vi "Instr_InitObject.vi"(8 "error in (no error)":errorcluster, 9 "Instrument Configuration":variant, 10 "GPIB Address":string, 11 "LXIPXISwitching in":refnum<class "LXIPXISwitching.lvclass">) -> (0 "error out":errorcluster, 3 "LXIPXISwitching out":refnum<class "LXIPXISwitching.lvclass">)   [LabVIEW 2018, in "LXIPXISwitching.lvclass"]
uses:
  LXIPXISwitching.lvclass
  LXIPXISwitching.lvclass/LXIPXISwitching.ctl
  InstrumentSetup.vi
  InstrControl.lvclass
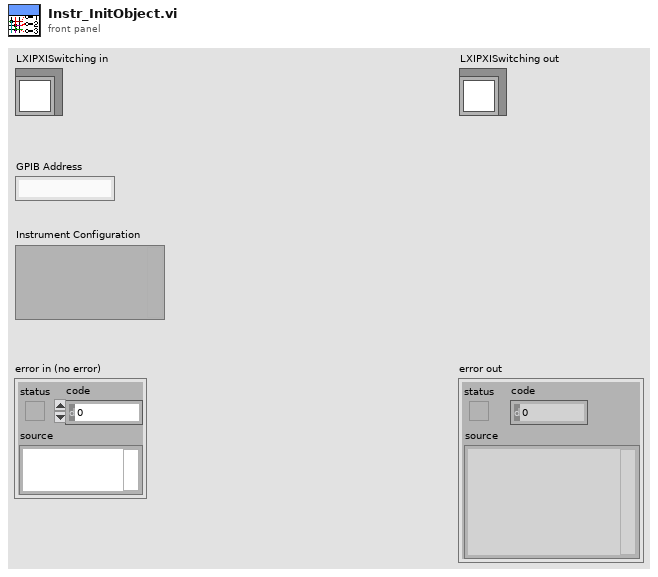
[diagram p1: front panel]
types:
  T1 = cluster{"MUX ":string, "Matrix":string, "Breadboard":string, "MUX  PN":string, "Matrix PN":string, "Breadboard PN":string}
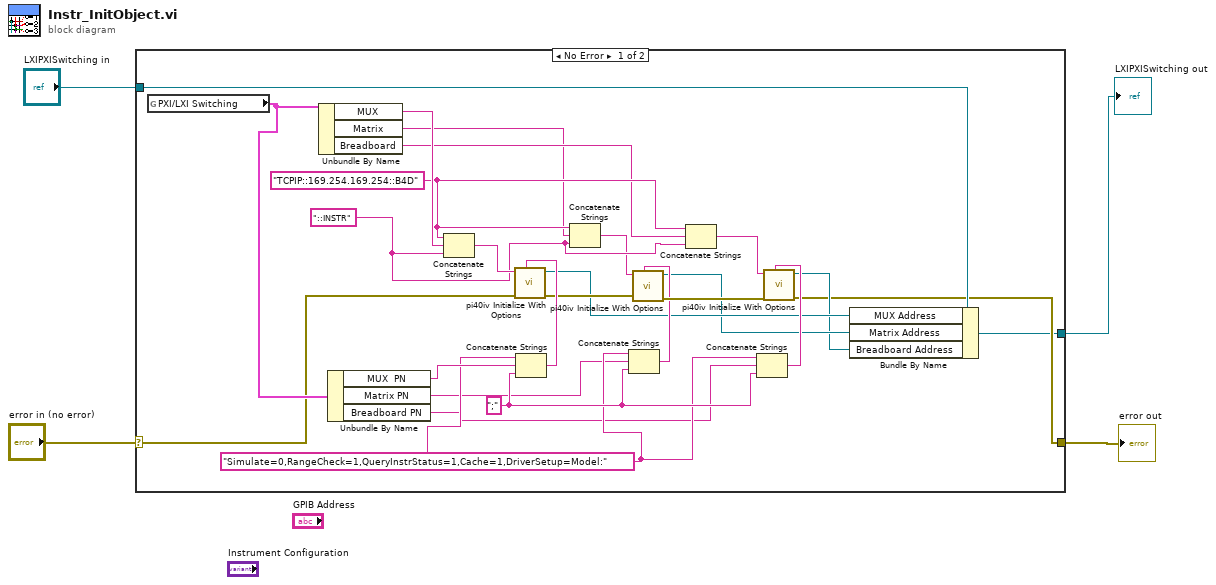
[diagram p0: block diagram]
diagram:
  n1 = case shown="No Error" "error in (no error)" {
    selector: "error in (no error)" -> [w25 w32]
    tunnel: [w6 w32] -> w3
    tunnel: "LXIPXISwitching in" -> [w10 w31]
    tunnel: [w5 w31] -> w1
    frame No Error {
      w16 = ";" ("string")
      w15 = "Simulate=0,RangeCheck=1,QueryInstrStatus=1,Cache=1,DriverSetup=Model:" ("option string")
      w22 = "TCPIP::169.254.169.254::B4D" ("string")
      w19 = "::INSTR" ("string")
      n2 = global read "InstrumentSetup.vi" "PXI/LXI Switching"() -> (w28:T1)
      n3 = Unbundle By Name(w28) -> ("MUX"=w30:string, "Matrix"=w20:string, "Breadboard"=w21:string)
      n4 = Unbundle By Name(w28) -> ("MUX  PN"=w27:string, "Matrix PN"=w14:string, "Breadboard PN"=w13:string)
      n5 = Concatenate Strings(w22, w30, w19) -> (w29:string)
      n6 = Concatenate Strings(w15, w27, w16) -> (w26:string)
      n7 = call <instrlib>:"pi40iv Initialize With Options.vi"("option string"=w26, "error in (no error)"=w25, "resource name"=w29) -> ("error out"=w24:errorcluster, "instrument handle out"=w9:refnum<k15>)  [unwired: 7 in]
      n8 = Concatenate Strings(w22, w20, w19) -> (w18:string)
      n9 = Concatenate Strings(w15, w14, w16) -> (w12:string)
      n10 = call <instrlib>:"pi40iv Initialize With Options.vi"("option string"=w12, "error in (no error)"=w24, "resource name"=w18) -> ("error out"=w23:errorcluster, "instrument handle out"=w8:refnum<k15>)  [unwired: 7 in]
      n11 = Concatenate Strings(w22, w21, w19) -> (w17:string)
      n12 = Concatenate Strings(w15, w13, w16) -> (w11:string)
      n13 = call <instrlib>:"pi40iv Initialize With Options.vi"("option string"=w11, "error in (no error)"=w23, "resource name"=w17) -> ("error out"=w6:errorcluster, "instrument handle out"=w7:refnum<k15>)  [unwired: 7 in]
      n14 = Bundle By Name(cluster=w10, "MUX Address"=w9, "Matrix Address"=w8, "Breadboard Address"=w7) -> (w5:refnum<class "LXIPXISwitching.lvclass">)
    }
    frame Error {
    }
  }
  "error out" <- w3
  "LXIPXISwitching out" <- w1
